vi "ExSubROIQ.vi"(2 "error in (no error)":errorcluster, 3 "ROI":T1={"X Start"=1, "X End"=1, "X Bin"=1, "Y Start"=1, "Y End"=1, "Y Bin"=1} {"Y Bin" min=1 step=1; "Y End" min=1 step=1; "Y Start" min=1 step=1; "X Bin" min=1 step=1; "X End" min=1 step=1; "X Start" min=1 step=1}, 4 "Camera Handle":u32) -> (0 "error out":errorcluster, 1 "Camera Handle":u32)   [LabVIEW 2010]
panel:
  # "ExSubROI:\nThis Sub-VI takes a ROI cluster and \nprograms up the camera using that\nROI."
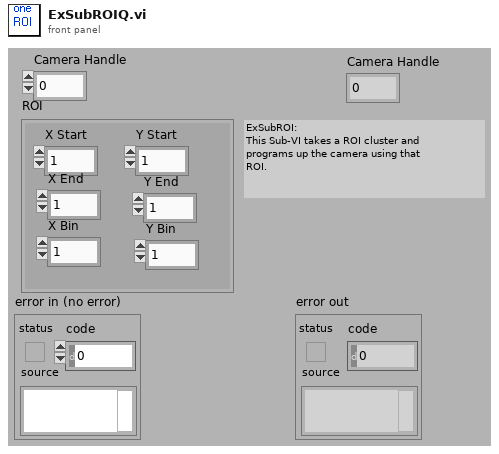
[diagram p1: front panel]
types:
  T1 = cluster{"X Start":u32, "X End":u32, "X Bin":u32, "Y Start":u32, "Y End":u32, "Y Bin":u32}
  T2 = cluster{"X start":u32, "X end":u32, "X Binning/Grouping":u32, "Y start":u32, "Y end":u32, "Y Binning/Grouping":u32}
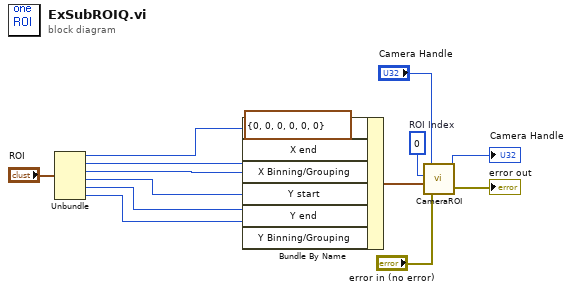
[diagram p0: block diagram]
diagram:
  w11 = u32 0  # ROI Index
  n1 = Unbundle("ROI") -> ("X Start"=w8:u32, "X End"=w1:u32, "X Bin"=w2:u32, "Y Start"=w3:u32, "Y End"=w4:u32, "Y Bin"=w5:u32)
  n2 = Bundle By Name(cluster=T2 {"X start"=0, "X end"=0, "X Binning/Grouping"=0, "Y start"=0, "Y end"=0, "Y Binning/Grouping"=0} ("ROI Params"), "X start"=w8, "X end"=w1, "X Binning/Grouping"=w2, "Y start"=w3, "Y end"=w4, "Y Binning/Grouping"=w5) -> (w10:T2)
  n3 = call <userlib>:"CameraROI.vi"("error in"="error in (no error)", "ROI Params"=w10, "ROI Index"=w11, "Camera Handle"="Camera Handle") -> ("error out"=→"error out":errorcluster, "Camera Handle"=→"Camera Handle":u32)
